vi "Measurement Parser.vi"(7 "Waveform Graph":dynamicdata(graph), 8 "error in (no error)":errorcluster, 9 "Generic Instrument.lvlib:Generic Card.lvclass":refnum<class "Generic Card.lvclass">, 10 "Data Array":dbl[](array[numeric]), 11 "Yokogawa WT1600 in":refnum<class "Yokogawa WT1600.lvclass">) -> (0 "error out":errorcluster, 3 "Yokogawa WT1600 out":refnum<class "Yokogawa WT1600.lvclass">)   [LabVIEW 2014, in "Generic Power Analyzer.lvlib" / "Yokogawa WT1600.lvlib" / "Yokogawa WT1600.lvclass"]
uses:
  Yokogawa WT1600.lvclass
  Generic Instrument/Generic Card/Generic Card.lvclass
  Universal Power Meter/Measured Value Header Control.ctl
  Generic Instrument/Generic Card/Generic Card.lvclass/Generic Card.ctl
  Generic Power Analyzer/Generic Power Analyzer.lvclass
  Data Logger/Data Logger.lvclass
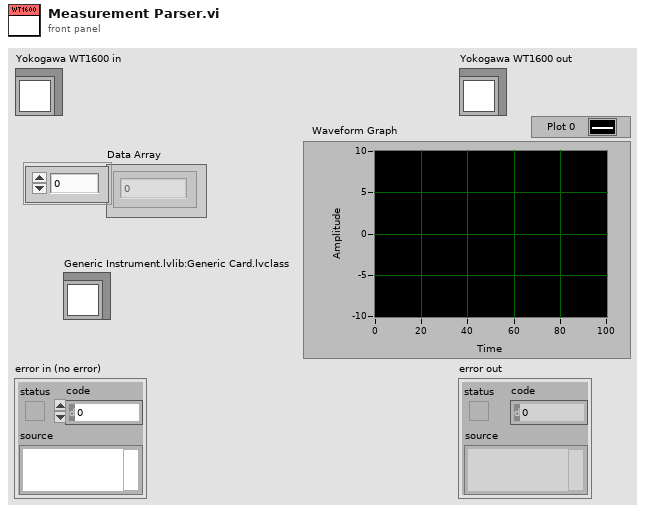
[diagram p1: front panel]
types:
  T1 = typedef "Measured Value Header Control.ctl" = enum16{"Power factor", "Current THD (%)", "Voltage THD (%)", "Amp-Hours", "Energy (Watt-hours)", "Frequency (Herts)", "Power (watts)", "Current RMS (amps)", "Voltage RMS (volts)"}
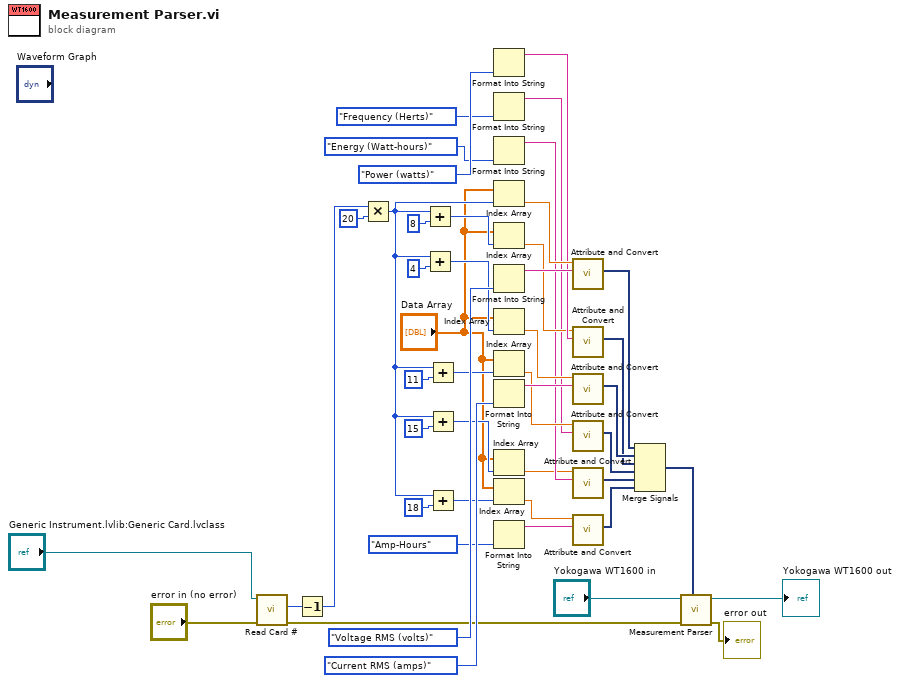
[diagram p0: block diagram]
diagram:
  n1 = call "Read Card #.vi"("error in (no error)"="error in (no error)", "Generic Card in"="Generic Instrument.lvlib:Generic Card.lvclass") -> ("error out"=w4:errorcluster, "Card #"=w45:u8)  [unwired: 7 in, 1 out]
  n2 = Decrement(x=w45) -> (x-1=w42:u8)
  n3 = Multiply(x=w42, y=u8 20) -> (x*y=w16:u8)
  n4 = Add(x=w16, y=u8 8) -> (x+y=w15:u8)
  n5 = Add(x=w16, y=u8 4) -> (x+y=w21:u8)
  n6 = Add(x=w16, y=u8 11) -> (x+y=w14:u8)
  n7 = Add(x=w16, y=u8 15) -> (x+y=w13:u8)
  n8 = Add(x=w16, y=u8 18) -> (x+y=w12:u8)
  n9 = Format Into String(Measured_Value_Header_Control."Power (watts)" ("Strings")) -> (resulting string=w36:string)  [unwired: 3 in, 1 out]
  n10 = Format Into String(Measured_Value_Header_Control."Frequency (Herts)" ("Strings")) -> (resulting string=w31:string)  [unwired: 3 in, 1 out]
  n11 = Format Into String(Measured_Value_Header_Control."Energy (Watt-hours)" ("Strings")) -> (resulting string=w30:string)  [unwired: 3 in, 1 out]
  n12 = Index Array(array="Data Array", index=w16) -> (element=w40:dbl)
  n13 = Index Array(array="Data Array", index=w15) -> (element=w34:dbl)
  n14 = Format Into String(Measured_Value_Header_Control."Voltage RMS (volts)" ("Strings")) -> (resulting string=w44:string)  [unwired: 3 in, 1 out]
  n15 = Index Array(array="Data Array", index=w21) -> (element=w39:dbl)
  n16 = Index Array(array="Data Array", index=w14) -> (element=w33:dbl)
  n17 = Format Into String(Measured_Value_Header_Control."Current RMS (amps)" ("Strings")) -> (resulting string=w37:string)  [unwired: 3 in, 1 out]
  n18 = Index Array(array="Data Array", index=w13) -> (element=w28:dbl)
  n19 = Index Array(array="Data Array", index=w12) -> (element=w25:dbl)
  n20 = Format Into String(Measured_Value_Header_Control."Amp-Hours" ("Strings")) -> (resulting string=w23:string)  [unwired: 3 in, 1 out]
  n21 = call "Attribute and Convert.vi"("Signal Name"=w44, "Number in"=w40) -> ("Dynamic Signal Out"=w27:dynamicdata)  [unwired: 9 in]
  n22 = call "Attribute and Convert.vi"("Signal Name"=w36, "Number in"=w34) -> ("Dynamic Signal Out"=w11:dynamicdata)  [unwired: 9 in]
  n23 = call "Attribute and Convert.vi"("Signal Name"=w37, "Number in"=w39) -> ("Dynamic Signal Out"=w26:dynamicdata)  [unwired: 9 in]
  n24 = call "Attribute and Convert.vi"("Signal Name"=w31, "Number in"=w33) -> ("Dynamic Signal Out"=w10:dynamicdata)  [unwired: 9 in]
  n25 = call "Attribute and Convert.vi"("Signal Name"=w30, "Number in"=w28) -> ("Dynamic Signal Out"=w9:dynamicdata)  [unwired: 9 in]
  n26 = call "Attribute and Convert.vi"("Signal Name"=w23, "Number in"=w25) -> ("Dynamic Signal Out"=w8:dynamicdata)  [unwired: 9 in]
  n27 = Merge Signals(w27, w26, w11, w10, w9, w8) -> (w2:dynamicdata)
  n28 = call-parent "Measurement Parser.vi"("Waveform Graph"=w2, "error in (no error)"=w4, "Generic Power Analyzer in"="Yokogawa WT1600 in") -> ("error out"=→"error out":errorcluster, "Generic Power Analyzer out"=→"Yokogawa WT1600 out":refnum<class "Yokogawa WT1600.lvclass">)  [unwired: 7 in]
